vi "SC10_get_id2.vi"(8 "error in (no error)":errorcluster, 11 "VISA resource name":refnum<visa-resource-name>) -> (0 "error out":errorcluster, 2 "Model":string, 3 "VISA resource name out":refnum<visa-resource-name>)   [LabVIEW 2010]
panel:
  out "read buffer":string
  out "return count 2":u32
  out "return count":u32
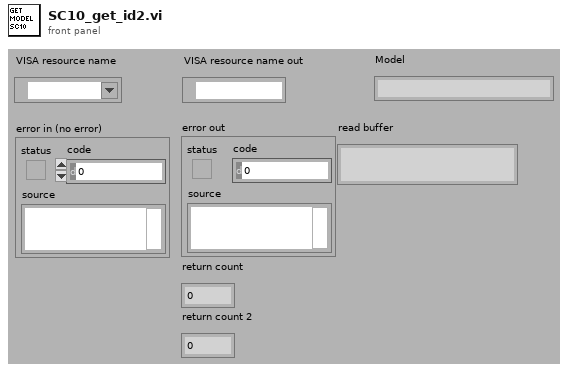
[diagram p1: front panel]
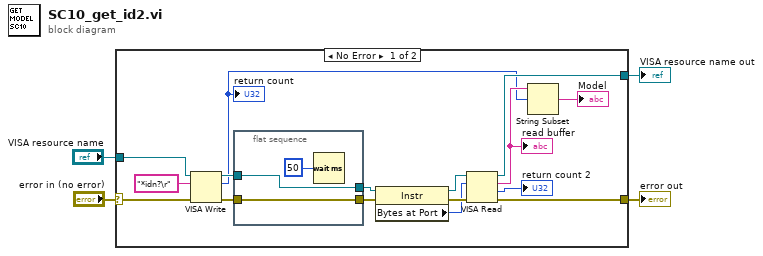
[diagram p0: block diagram]
diagram:
  n1 = case shown="No Error" "error in (no error)" {
    selector: "error in (no error)" -> [w18 w24]
    tunnel: [w17 w24] -> w3
    tunnel: [w14 w25] -> w2
    tunnel: "VISA resource name" -> [w13 w25]
    frame No Error {
      n2 = VISA Write(VISA resource name=w13, write buffer="*idn?\r", error in (no error)=w18) -> (VISA resource name out=w20:refnum<visa-resource-name>, return count=w10:u32, error out=w19:errorcluster)
      "return count" <- w10
      n3 = flat-sequence {
        tunnel: w20 -> [w22]
        tunnel: [w22] -> w9
        tunnel: w19 -> [w21]
        tunnel: [w21] -> w8
        frame #0 {
          n4 = Wait (ms)(milliseconds to wait=u32 50) -> ()  [unwired: 1 out]
        }
      }
      n5 = property class="Instr"(reference=w9, error in=w8) -> (reference out=w6:refnum<visa-resource-name>, error out=w7:errorcluster, "Bytes at Port"=w5:u32)
      n6 = VISA Read(VISA resource name=w6, byte count=w5, error in (no error)=w7) -> (VISA resource name out=w14:refnum<visa-resource-name>, read buffer=w12:string, return count=→"return count 2":u32, error out=w17:errorcluster)
      "read buffer" <- w12
      n7 = String Subset(string=w12, offset (0)=w10) -> (substring=→"Model":string)  [unwired: 1 in]
    }
    frame Error {
    }
  }
  "error out" <- w3
  "VISA resource name out" <- w2
